vi "Wait.vi"(8 "error In":errorcluster, 11 "Wait Time In":u32) -> (0 "error Out":errorcluster)   [LabVIEW 2015]
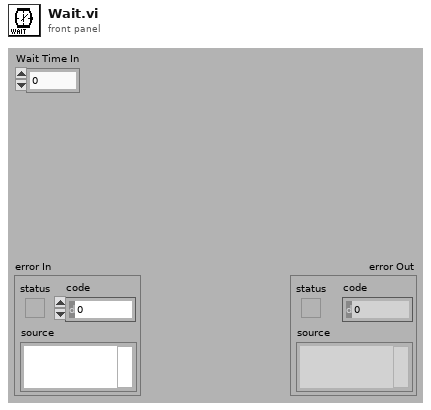
[diagram p1: front panel]
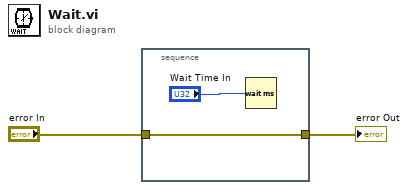
[diagram p0: block diagram]
diagram:
  n1 = stacked-sequence {
    tunnel: "error In" -> [w3]
    tunnel: [w3] -> w1
    frame #0 {
      n2 = Wait (ms)(milliseconds to wait="Wait Time In") -> ()  [unwired: 1 out]
    }
  }
  "error Out" <- w1
